vi "SR_J-Check Steering Input.vi"(8 "error in (no error)":errorcluster, 10 "RDS Message":refnum<user-event>, 11 "Joystick":T1) -> (0 "error out":errorcluster, 2 "RDS Message out":refnum<user-event>, 3 "Joystick 2":T1)   [LabVIEW 2015, in "Shore Library.lvlib"]
uses:
  Shore Library.lvlib
  Libraries/RDS Framework/RDS Message Class/RDS Message.lvclass
  SR-J-State.ctl
  Libraries/RDS Child Messages/Helm/Steering Command/Steering Command Cntrl.ctl
  Libraries/RDS Child Messages/RDS Child Messages.lvlib
  Libraries/Geo/RDS Libraries.lvlib
  Actors/RDS Helm Actor/RDS Helm Actor.lvlib
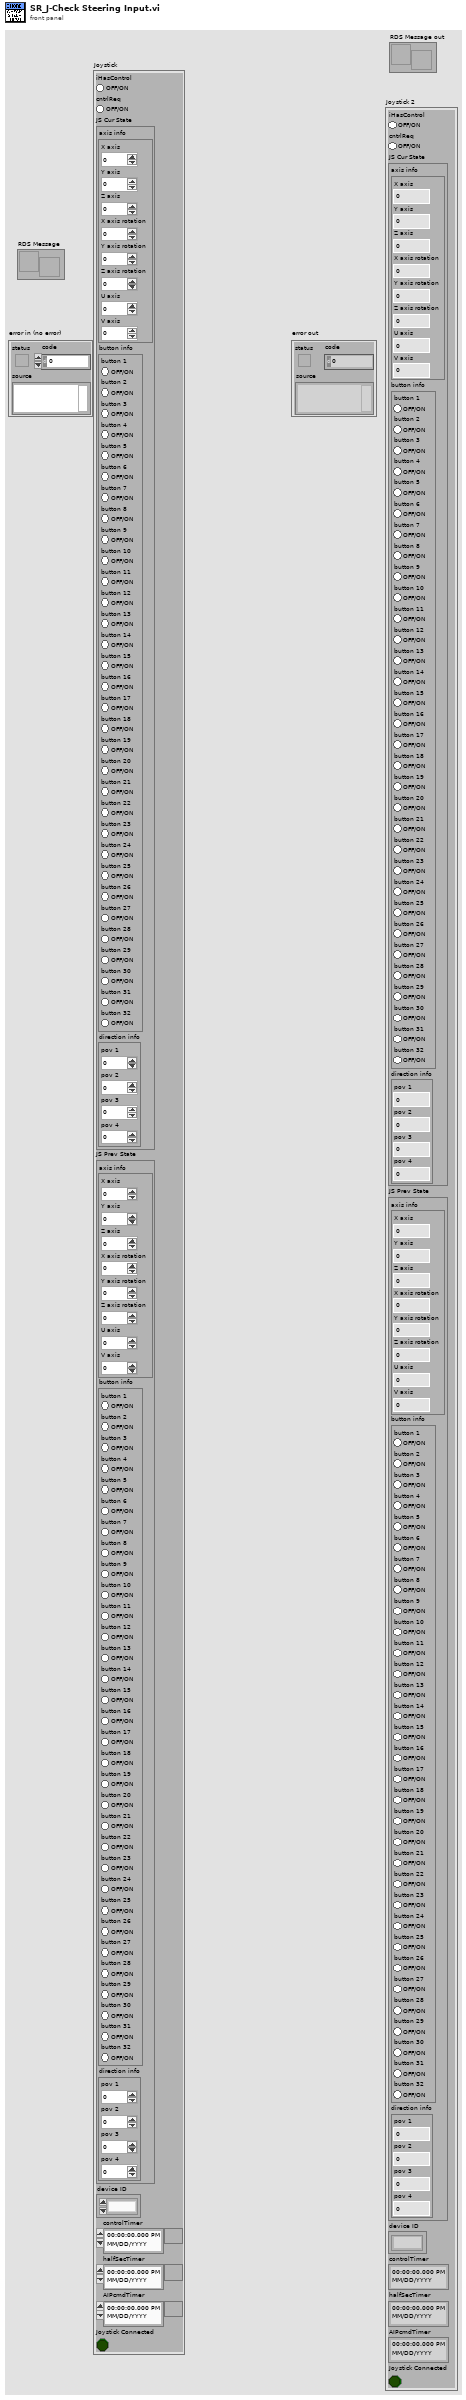
[diagram p1: front panel]
types:
  T1 = typedef "Shore Library.lvlib/SR-J-State.ctl" = cluster{"iHasControl":bool, "cntrlReq":bool, "JS Cur State":cluster{"axis info":cluster{"X axis":i32, "Y axis":i32, "Z axis":i32, "X axis rotation":i32, "Y axis rotation":i32, "Z axis rotation":i32, "U axis":i32, "V axis":i32}, "button info":cluster{"button 1":bool, "button 2":bool, "button 3":bool, "button 4":bool, "button 5":bool, "button 6":bool, "button 7":bool, "button 8":bool, "button 9":bool, "button 10":bool, "button 11":bool, "button 12":bool, "button 13":bool, "button 14":bool, "button 15":bool, "button 16":bool, "button 17":bool, "button 18":bool, "button 19":bool, "button 20":bool, "button 21":bool, "button 22":bool, "button 23":bool, "button 24":bool, "button 25":bool, "button 26":bool, "button 27":bool, "button 28":bool, "button 29":bool, "button 30":bool, "button 31":bool, "button 32":bool}, "direction info":cluster{"pov 1":i32, "pov 2":i32, "pov 3":i32, "pov 4":i32}}, "JS Prev State":cluster{"axis info":cluster{"X axis":i32, "Y axis":i32, "Z axis":i32, "X axis rotation":i32, "Y axis rotation":i32, "Z axis rotation":i32, "U axis":i32, "V axis":i32}, "button info":cluster{"button 1":bool, "button 2":bool, "button 3":bool, "button 4":bool, "button 5":bool, "button 6":bool, "button 7":bool, "button 8":bool, "button 9":bool, "button 10":bool, "button 11":bool, "button 12":bool, "button 13":bool, "button 14":bool, "button 15":bool, "button 16":bool, "button 17":bool, "button 18":bool, "button 19":bool, "button 20":bool, "button 21":bool, "button 22":bool, "button 23":bool, "button 24":bool, "button 25":bool, "button 26":bool, "button 27":bool, "button 28":bool, "button 29":bool, "button 30":bool, "button 31":bool, "button 32":bool}, "direction info":cluster{"pov 1":i32, "pov 2":i32, "pov 3":i32, "pov 4":i32}}, "device ID":refnum<k1>, "controlTimer":timestamp, "halfSecTimer":timestamp, "AIPcmdTimer":timestamp, "Joystick Connected":bool}
  T2 = typedef "RDS Child Messages.lvlib/Steering Command Cntrl.ctl" = cluster{"Throttle":i16, "Rudder":i8, "Duration (s)":u16}
  T3 = cluster{"axis info":cluster{"X axis":i32, "Y axis":i32, "Z axis":i32, "X axis rotation":i32, "Y axis rotation":i32, "Z axis rotation":i32, "U axis":i32, "V axis":i32}, "button info":cluster{"button 1":bool, "button 2":bool, "button 3":bool, "button 4":bool, "button 5":bool, "button 6":bool, "button 7":bool, "button 8":bool, "button 9":bool, "button 10":bool, "button 11":bool, "button 12":bool, "button 13":bool, "button 14":bool, "button 15":bool, "button 16":bool, "button 17":bool, "button 18":bool, "button 19":bool, "button 20":bool, "button 21":bool, "button 22":bool, "button 23":bool, "button 24":bool, "button 25":bool, "button 26":bool, "button 27":bool, "button 28":bool, "button 29":bool, "button 30":bool, "button 31":bool, "button 32":bool}, "direction info":cluster{"pov 1":i32, "pov 2":i32, "pov 3":i32, "pov 4":i32}}
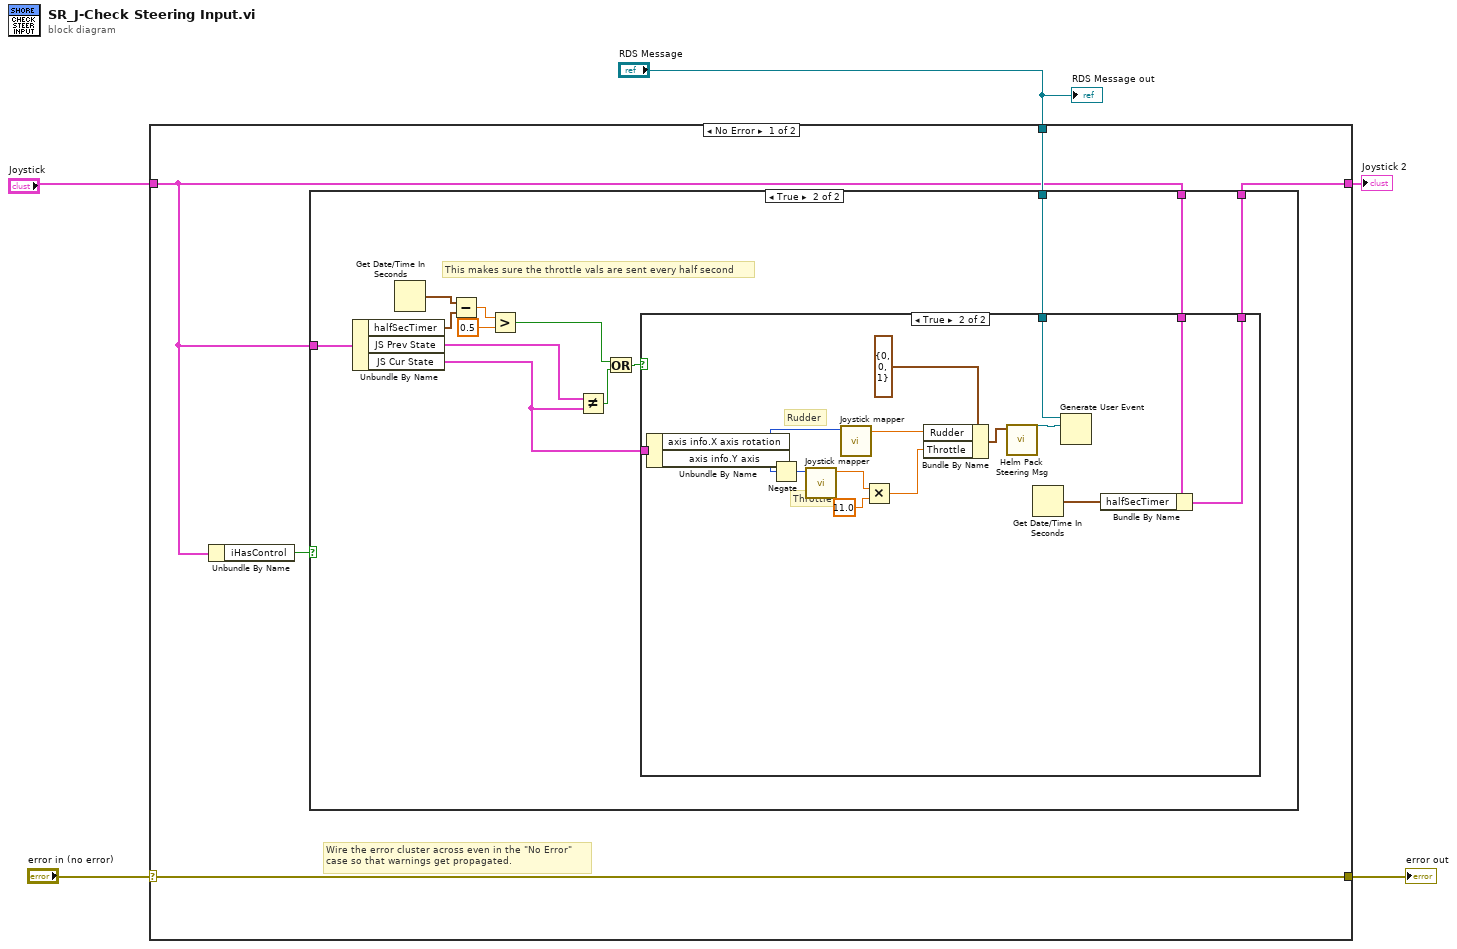
[diagram p0: block diagram]
diagram:
  n1 = case shown="No Error" "error in (no error)" {
    selector: "error in (no error)" -> [w10 w42]
    tunnel: [w10 w42] -> w4
    tunnel: [w8 w41] -> w1
    tunnel: "Joystick" -> [w6 w41]
    tunnel: "RDS Message" -> [w7 _]
    frame No Error {
      # "Wire the error cluster across even in the \"No Error\"\ncase so that warnings get propagated."
      n2 = Unbundle By Name(w6) -> ("iHasControl"=w9:bool)
      n3 = case shown="True" w9 {
        tunnel: w6 -> [_ w24]
        tunnel: w7 -> [_ w15]
        tunnel: [w11 w13] -> w8
        tunnel: w6 -> [w11 w12]
        frame False {
        }
        frame True {
          # "This makes sure the throttle vals are sent every half second"
          n4 = Unbundle By Name(w24) -> ("halfSecTimer"=w22:timestamp, "JS Prev State"=w23:T3, "JS Cur State"=w14:T3)
          n5 = Get Date/Time In Seconds() -> (seconds since 1Jan1904=w21:timestamp)
          n6 = Subtract(x=w21, y=w22) -> (x-y=w20:dbl)
          n7 = Greater?(x=w20, y=0.5) -> (0:w18:bool)
          n8 = Not Equal?(x=w23, y=w14) -> (x != y?=w17:bool)
          n9 = Or(x=w18, y=w17) -> (x .or. y?=w16:bool)
          n10 = case shown="True" w16 {
            tunnel: w14 -> [_ w40]
            tunnel: w15 -> [_ w27]
            tunnel: [w25 w32] -> w13
            tunnel: w12 -> [w25 w26]
            frame False {
            }
            frame True {
              # "Throttle"
              # "Rudder"
              n11 = Unbundle By Name(w40) -> ("axis info.X axis rotation"=w39:i32, "axis info.Y axis"=w38:i32)
              n12 = Negate(x=w38) -> (-x=w37:i32)
              n13 = call "Joystick mapper.vi"("Input"=w37) -> ("Output"=w30:dbl)  [unwired: 10 in]
              n14 = call "Joystick mapper.vi"("Input"=w39) -> ("Output"=w36:dbl)  [unwired: 10 in]
              n15 = Multiply(x=w30, y=11.0) -> (x*y=w29:dbl)
              n16 = Bundle By Name(cluster=T2 {"Throttle"=0, "Rudder"=0, "Duration (s)"=1} ("Steering Command Control"), "Rudder"=w36, "Throttle"=w29) -> (w34:T2)
              n17 = call "Helm Pack Steering Msg.vi"("Steering Command Control"=w34) -> ("Steer Msg"=w28:refnum<class "Steering Command.lvclass">)  [unwired: 9 in, 1 out]
              n18 = Get Date/Time In Seconds() -> (seconds since 1Jan1904=w33:timestamp)
              n19 = Generate User Event(user event=w27, event data cluster=w28) -> ()  [unwired: 2 in, 2 out]
              n20 = Bundle By Name(cluster=w26, "halfSecTimer"=w33) -> (w32:T1)
            }
          }
        }
      }
    }
    frame Error {
    }
  }
  "error out" <- w4
  "Joystick 2" <- w1
  "RDS Message out" <- "RDS Message"
